vi "ManufacturerInfo.vi"(8 "error in (no error)":errorcluster, 11 "new reference":refnum<k24>) -> (0 "error out":errorcluster, 3 "VGS_ManufacturerInfo out":refnum<class "VGS_ManufacturerInfo.lvclass">)   [LabVIEW 2022 SP3, in "LV_VGS.lvlib" / "VGS_ManufacturerInfo.lvclass"]
uses:
  VGS_ManufacturerInfo.lvclass
  C:/Users/Andrey/Documents/GitHub/LV_VGS/vgs_project.dll
  vgs_project.dll
  VGS_ManufacturerInfo.lvclass/VGS_ManufacturerInfo.ctl
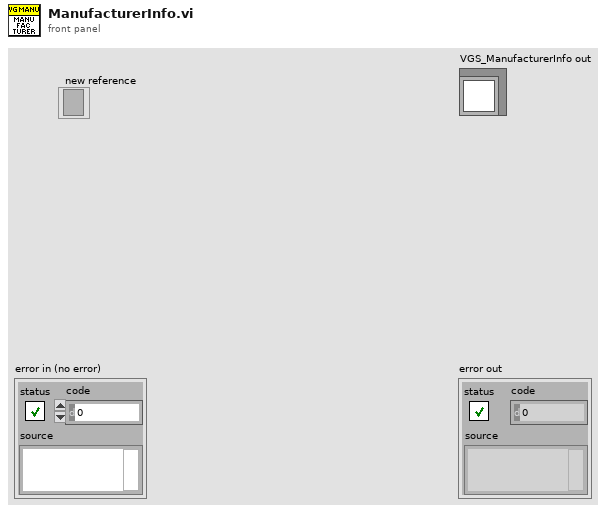
[diagram p1: front panel]
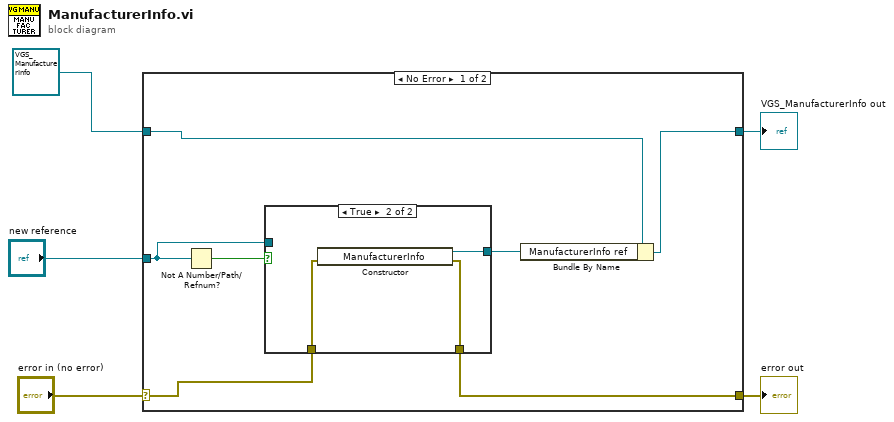
[diagram p0: block diagram]
diagram:
  n1 = case shown="No Error" "error in (no error)" {
    selector: "error in (no error)" -> [w9 w19]
    tunnel: [w8 w19] -> w4
    tunnel: [w11 w18] -> w2
    tunnel: refnum<class "VGS_ManufacturerInfo.lvclass"> refnum ("VGS_ManufacturerInfo in") -> [w12 w18]
    tunnel: "new reference" -> [w6 _]
    frame No Error {
      n2 = Not A Number/Path/Refnum?(number/path/refnum=w6) -> (NaN/Path/Refnum?=w7:bool)
      n3 = case shown="True" w7 {
        tunnel: [w14 w17] -> w10
        tunnel: w9 -> [w13 w16]
        tunnel: [w13 w15] -> w8
        tunnel: w6 -> [w14 _]
        frame False {
        }
        frame True {
          n4 = constructor class="ManufacturerInfo"(error in=w16) -> (reference out=w17:refnum<k24>, error out=w15:errorcluster)  [unwired: 2 in, 1 out]
        }
      }
      n5 = Bundle By Name(cluster=w12, "ManufacturerInfo ref"=w10) -> (w11:refnum<class "VGS_ManufacturerInfo.lvclass">)
    }
    frame Error {
    }
  }
  "error out" <- w4
  "VGS_ManufacturerInfo out" <- w2
